vi "FTS Get Acquisition Option Single Gain Level.vi"(7 "channel":u16, 8 "error in (no error)":errorcluster, 11 "specIndex":u16) -> (0 "error out":errorcluster, 3 "function return":i32)   [LabVIEW 2010, in "FTSLib.lvlib"]
doc: "int __cdecl FTS_GetAcquisitionOption_SingleGainLevel(unsigned short specIndex);"
uses:
  FTSLib.lvlib
  FTSLib.dll
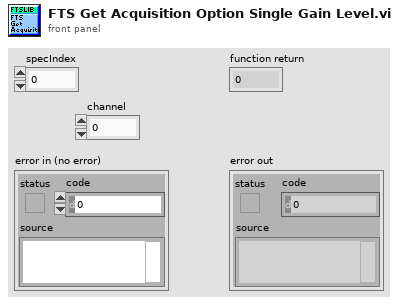
[diagram p1: front panel]
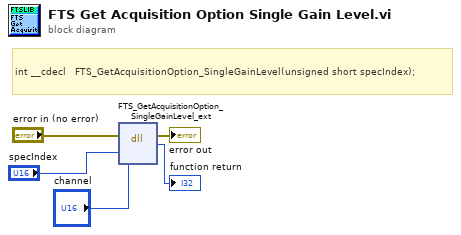
[diagram p0: block diagram]
diagram:
  # "int __cdecl   FTS_GetAcquisitionOption_SingleGainLevel(unsigned short specIndex);"
  n1 = dll-call lib="FTSLib.*" fn="FTS_GetAcquisitionOption_SingleGainLevel_ext"(error in="error in (no error)", "specIndex"="specIndex", "channel"="channel") -> (error out=→"error out":errorcluster, "return type"=→"function return":i32)  [unwired: 4 in, 1 out]
